vi "TEST - Is One Frontmost.vi"(8 "error in (no error)":errorcluster) -> (0 "error out":errorcluster, 2 "pass":bool)   [LabVIEW 2020]
uses:
  <userlib>/_OpenG.lib/error/error.llb/openg_error.lvlib
  <userlib>/_OpenG.lib/string/string.llb/openg_string.lvlib
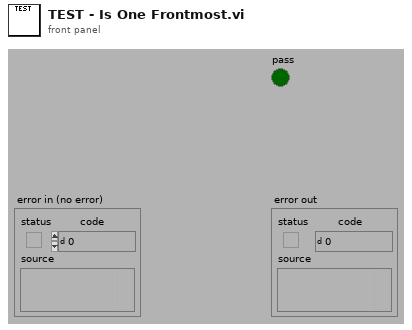
[diagram p1: front panel]
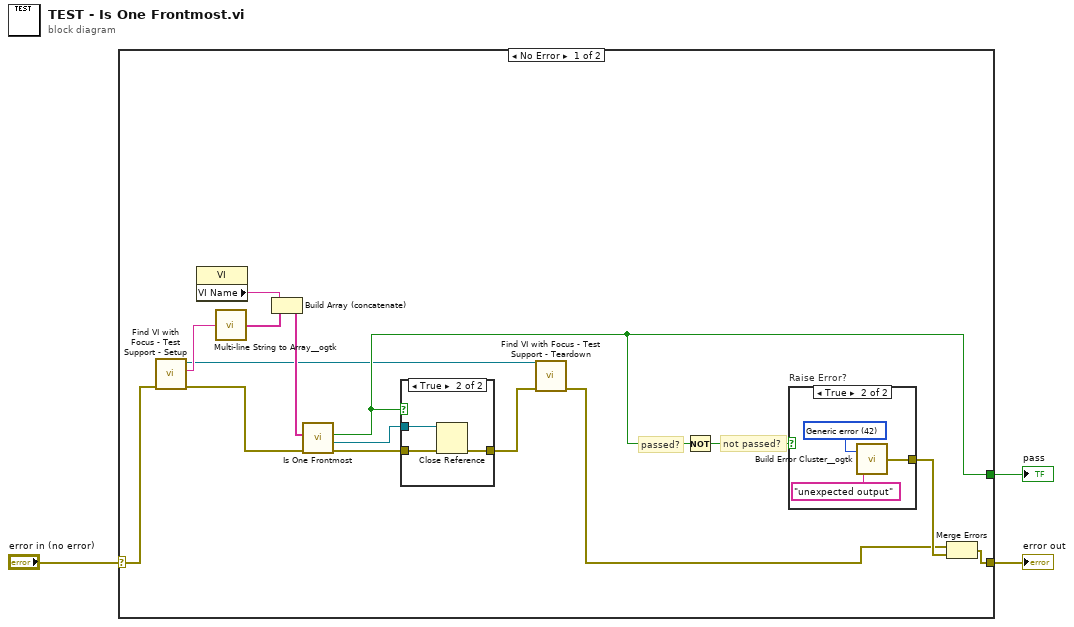
[diagram p0: block diagram]
diagram:
  n1 = case shown="No Error" "error in (no error)" {
    selector: "error in (no error)" -> [w8 w26]
    tunnel: [w11 _] -> w3
    tunnel: [w18 w26] -> w1
    frame No Error {
      # "not passed?"
      # "passed?"
      n2 = call "Find VI with Focus - Test Support - Setup.vi"("error in (no error)"=w8) -> ("error out"=w7:errorcluster, "VI Name"=w10:string, "VI Renum"=w9:refnum<vi>)  [unwired: 8 in]
      n3 = property class="VI"() -> ("VI Name"=w15:string)  [unwired: 2 in, 2 out]
      n4 = call <userlib>:"Multi-line String to Array__ogtk.vi"("string"=w10) -> ("lines"=w14:string[])
      n5 = Build Array (concatenate)(w15, w14) -> (w12:string[])
      n6 = call "Is One Frontmost.vi"("error in"=w7, "VI names"=w12) -> ("error out"=w6:errorcluster, "VI Refnum"=w13:refnum<vi>, "yes"=w11:bool)  [unwired: 6 in, 1 out]
      n7 = case shown="True" w11 {
        tunnel: w13 -> [_ w22]
        tunnel: w6 -> [w19 w21]
        tunnel: [w19 w20] -> w4
        frame False {
        }
        frame True {
          n8 = Close Reference(reference=w22, error in (no error)=w21) -> (error out=w20:errorcluster)
        }
      }
      n9 = call "Find VI with Focus - Test Support - Teardown.vi"("error in (no error)"=w4, "VI Renum"=w9) -> ("error out"=w5:errorcluster)  [unwired: 9 in]
      n10 = Not(x=w11) -> (.not. x?=w16:bool)
      n11 = case "Raise Error?" shown="True" w16 {
        tunnel: [_ w23] -> w17
        frame False {
        }
        frame True {
          w24 = 42 items=["No error", "Argument error", "Memory is full", "Out of zone", "End of file", "File already open", "Generic file I/O error", "File not found", "File permission error", "Disk is full", "Duplicate path", "Too many files open", "System feature not enabled", "Resource file not found", "Cannot add resource", "Resource not found", "Image not found", "Image memory error", "Pen does not exist", "Config type invalid", "Config token not found", "Config parse error", "Config memory error", "Bad external code format", "Bad external code offset", "External code not present", "Null window", "Destroy window error", "Null menu", "Print aborted", "Bad print record", "Print driver error", "Windows error during printing", "Memory error during printing", "Print dialog error", "Generic print error", "Invalid device refnum", "Device not found", "Device parameter error", "Device unit error", "Cannot open device", "Device call aborted", "Generic error", "Cancelled by user", "Object ID too low", "Object ID too high", "Object not in heap", "Unknown heap", "Unknown object (invalid DefProc)", "Unknown object (DefProc not in table)", "Message out of range", "Invalid (null) method", "Unknown message", "Manager call not supported", "Bad address", "Network operation in progress", "Network operation timed out", "Connection is busy", "Network attribute not supported", "Network error", "Address in use", "System out of memory", "Connection aborted", "Connection refused", "Not connected", "Already connected", "Connection closed", "Initialization error (interapplication manager)", "Bad occurrence", "Wait on unbound occurrence handler", "Occurrence queue overflow", "Datalog type conflict", "Unused", "Unrecognized type (interapplication manager)", "Memory corrupt", "Failed to make temporary DLL", "Old CIN version", "Drag socket not found", "Failed to load drop-object", "Failed to register OLE object", "Failed to release OLE object", "Format specifier type mismatch", "Unknown format specifier", "Too few format specifiers", "Too many format specifiers", "Scan failed", "Newer CIN version", "Error converting to variant", "Runtime menu error", "Password tampered", "Variant attribute not found", "Incompatible variant data type", "Event data is not available", "Event Store is not present", "Occurrence is not found", "Event Queue is not created", "Event info is not available", "Refnum passed is NULL", "Error retrieving Class GUID", "Error retrieving CoClass GUID", "Error retrieving TypeLib GUID.", "Bad built application magic bytes.", "Specific driver is different from the specific driver associated with the Logical Name.", "There is no session opened to the class driver.", "Max Error", "MAX - Error with config objects", "MAX - Error loading configuration", "MAX - Group not supported"]
          n12 = call <userlib>:"Build Error Cluster__ogtk.vi"("String to Prepend to source (\"\")"="unexpected output" ("String to Prepend to source (\"\")"), "code"=w24) -> ("error out"=w23:errorcluster)
        }
      }
      n13 = Merge Errors(w5, w17) -> (w18:errorcluster)
    }
    frame Error {
    }
  }
  "pass" <- w3
  "error out" <- w1
